vi "CLD 7 Time Stamp to Initialization String Solution.vi"(8 "Error In":errorcluster) -> (0 "Error Out":errorcluster, 3 "Code String Out":string)   [LabVIEW 2018]
doc: "CLD 7: The additional indicators are used for troubleshooting. \n\nFor solutions using non-US time stamps the parsing will be slightly different. This solution is made for a US time stamp, and a switch provides two strings that would be produced by a US time stamp."
panel:
  in  "Switch T = International, F = US time stamp":bool caption="International Switch"
  out "Year":string
  out "Date":string
  out "Month":string
  out "Day":string
  out "AM/PM":string
  out "Seconds":string
  out "Minutes":string
  out "Hour":string
  out "date string":string
  out "time string":string
  # "Indicators used for  troubleshooting below"
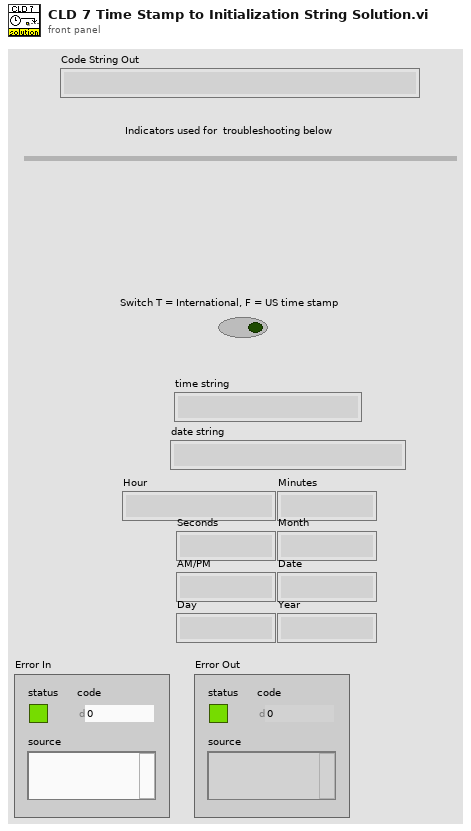
[diagram p1: front panel]
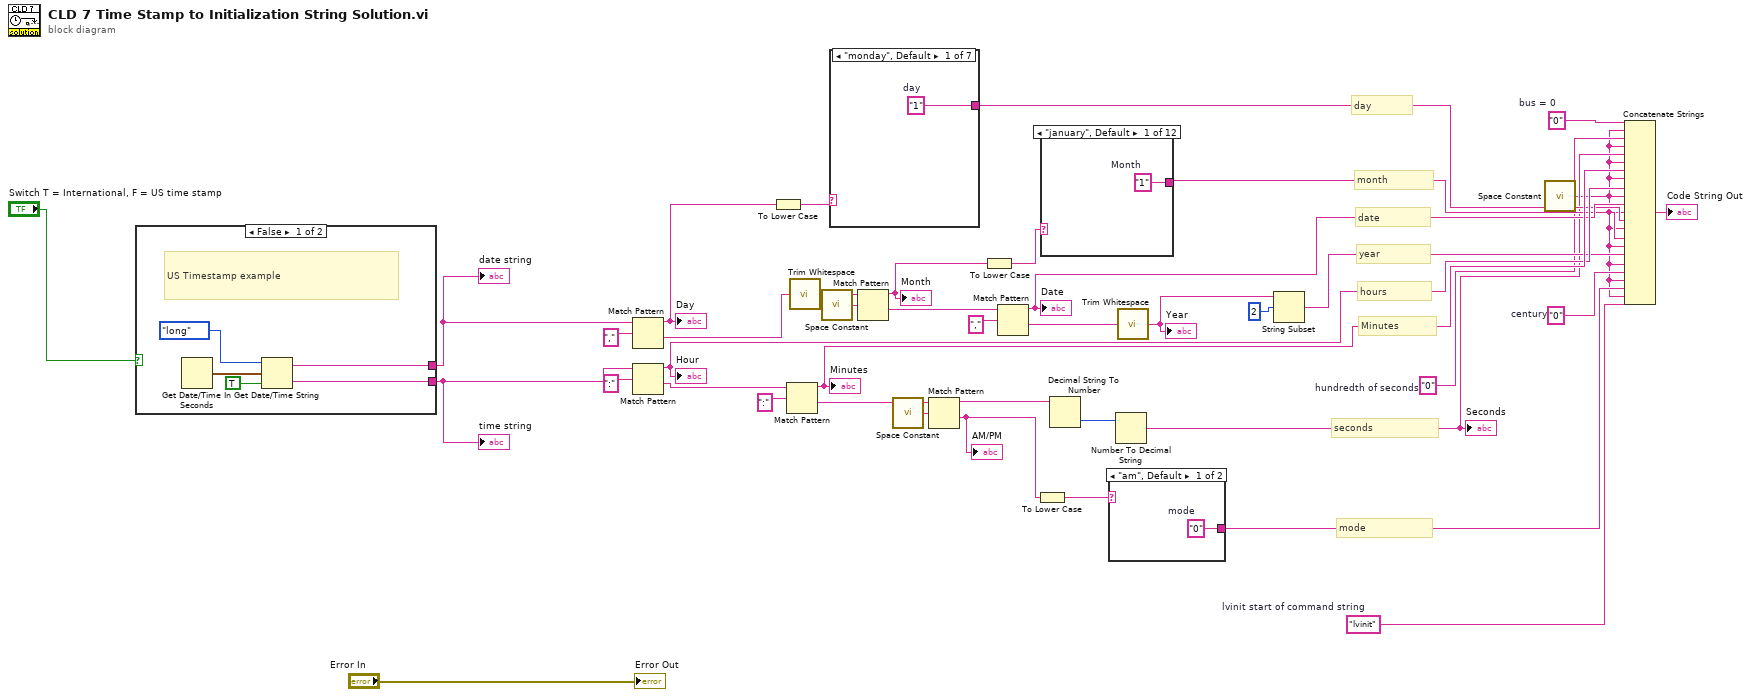
[diagram p0: block diagram]
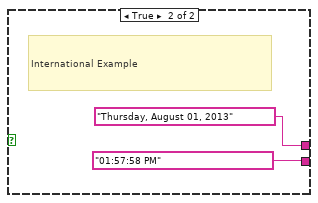
[diagram p2: hidden frame]
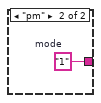
[diagram p3: hidden frame]
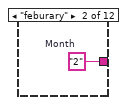
[diagram p4: hidden frame]
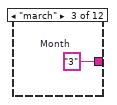
[diagram p5: hidden frame]
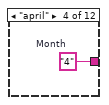
[diagram p6: hidden frame]
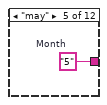
[diagram p7: hidden frame]
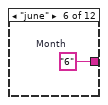
[diagram p8: hidden frame]
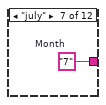
[diagram p9: hidden frame]
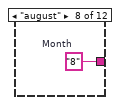
[diagram p10: hidden frame]
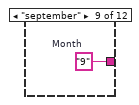
[diagram p11: hidden frame]
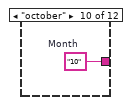
[diagram p12: hidden frame]
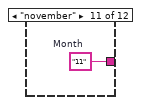
[diagram p13: hidden frame]
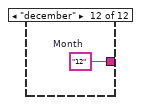
[diagram p14: hidden frame]
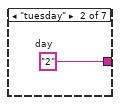
[diagram p15: hidden frame]
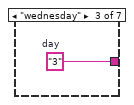
[diagram p16: hidden frame]
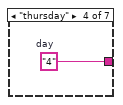
[diagram p17: hidden frame]
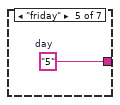
[diagram p18: hidden frame]
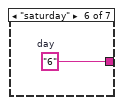
[diagram p19: hidden frame]
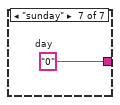
[diagram p20: hidden frame]
diagram:
  w7 = "0"  # bus = 0
  w14 = "0"  # century
  w3 = "0"  # hundredth of seconds
  w8 = "lvinit"  # lvinit start of command string
  # "Minutes"
  # "hours"
  # "date"
  # "day"
  # "month"
  # "year"
  # "mode"
  # "seconds"
  n1 = case shown="False" "Switch T = International, F = US time stamp" {
    tunnel: [w42 "01:57:58 PM"] -> w35
    tunnel: [w41 "Thursday, August 01, 2013"] -> w27
    frame False {
      # "US Timestamp example"
      n2 = Get Date/Time In Seconds() -> (seconds since 1Jan1904=w45:timestamp)
      n3 = Get Date/Time String(date format (0)=enum16{"short", "long", "abbreviated"}."long", seconds (now)=w45, want seconds? (F)=TRUE) -> (date string=w41:string, time string=w42:string)
    }
    frame True {
      # "International Example"
    }
  }
  "time string" <- w35
  "date string" <- w27
  n4 = Match Pattern(string=w27, regular expression=",") -> (before substring=w23:string, after substring=w33:string)  [unwired: 1 in, 2 out]
  "Day" <- w23
  n5 = Match Pattern(string=w35, regular expression=":") -> (before substring=w25:string, after substring=w38:string)  [unwired: 1 in, 2 out]
  "Hour" <- w25
  n6 = To Lower Case(string=w23) -> (all lower case string=w22:string)
  n7 = Match Pattern(string=w38, regular expression=":") -> (before substring=w26:string, after substring=w37:string)  [unwired: 1 in, 2 out]
  "Minutes" <- w26
  n8 = call <vilib>:"Trim Whitespace.vi"("string"=w33) -> ("trimmed string"=w32:string)  [unwired: 1 in]
  n9 = call <vilib>:"Space Constant.vi"() -> ("String"=w31:string)
  n10 = case shown="\"monday\", Default" w22 {
    tunnel: [w48 w49 w50 w51 w52 w53 w54] -> w21
    frame "monday", Default {
      w48 = "1"  # day
    }
    frame "tuesday" {
      w49 = "2"  # day
    }
    frame "wednesday" {
      w50 = "3"  # day
    }
    frame "thursday" {
      w51 = "4"  # day
    }
    frame "friday" {
      w52 = "5"  # day
    }
    frame "saturday" {
      w53 = "6"  # day
    }
    frame "sunday" {
      w54 = "0"  # day
    }
  }
  n11 = Match Pattern(string=w32, regular expression=w31) -> (before substring=w20:string, after substring=w29:string)  [unwired: 1 in, 2 out]
  "Month" <- w20
  n12 = call <vilib>:"Space Constant.vi"() -> ("String"=w36:string)
  n13 = Match Pattern(string=w37, regular expression=w36) -> (before substring=w5:string, after substring=w13:string)  [unwired: 1 in, 2 out]
  "AM/PM" <- w13
  n14 = To Lower Case(string=w20) -> (all lower case string=w19:string)
  n15 = Match Pattern(string=w29, regular expression=",") -> (before substring=w24:string, after substring=w28:string)  [unwired: 1 in, 2 out]
  "Date" <- w24
  n16 = To Lower Case(string=w13) -> (all lower case string=w12:string)
  n17 = case shown="\"january\", Default" w19 {
    tunnel: [w55 w56 w57 w58 w59 w60 w61 w62 w63 w64 w65 w66] -> w18
    frame "january", Default {
      w55 = "1"  # Month
    }
    frame "feburary" {
      w56 = "2"  # Month
    }
    frame "march" {
      w57 = "3"  # Month
    }
    frame "april" {
      w58 = "4"  # Month
    }
    frame "may" {
      w59 = "5"  # Month
    }
    frame "june" {
      w60 = "6"  # Month
    }
    frame "july" {
      w61 = "7"  # Month
    }
    frame "august" {
      w62 = "8"  # Month
    }
    frame "september" {
      w63 = "9"  # Month
    }
    frame "october" {
      w64 = "10"  # Month
    }
    frame "november" {
      w65 = "11"  # Month
    }
    frame "december" {
      w66 = "12"  # Month
    }
  }
  n18 = Decimal String To Number(string=w5) -> (number=w6:i32)  [unwired: 2 in, 1 out]
  n19 = case shown="\"am\", Default" w12 {
    tunnel: [w67 w68] -> w11
    frame "am", Default {
      w67 = "0"  # mode
    }
    frame "pm" {
      w68 = "1"  # mode
    }
  }
  n20 = Number To Decimal String(number=w6) -> (decimal integer string=w4:string)  [unwired: 1 in]
  "Seconds" <- w4
  n21 = call <vilib>:"Trim Whitespace.vi"("string"=w28) -> ("trimmed string"=w17:string)  [unwired: 1 in]
  "Year" <- w17
  n22 = String Subset(string=w17, offset (0)=2) -> (substring=w15:string)  [unwired: 1 in]
  n23 = call <vilib>:"Space Constant.vi"() -> ("String"=w2:string)
  n24 = Concatenate Strings(w7, w2, w3, w2, w4, w2, w26, w2, w25, w2, w24, w2, w21, w2, w18, w2, w15, w2, w14, w2, w11, w2, w8) -> (→"Code String Out":string)
  "Error Out" <- "Error In"
